vi "ColourSensorProcess.vi"(8 "error in (no error)":errorcluster, 9 "I2C Ref Out":T1={"myRIO Reference"={"myRIO Model"=enum."myRIO-1900", "myRIO Hardware Reference"={"Generic FPGA Reference"=refnum, "Allow multiple opens"=TRUE}}, "I2C Channels Enum"=enum."A/I2C", "I2C Configuration"={"I2C Transfer Rate"=enum."Fast mode (400 kbps)"}}, 10 "Just the ascending angles":dbl[](array[numeric])=[0.0, 0.49085178039801924, 0.49085178039801924, 0.4969686048790533, 0.5016040541891205, 0.5028432109278608, 0.5084893240796899, 0.5084893240796899, 0.5084893240796899, 0.5084893240796899, 0.5115561271703055, 0.5123894603107377, 0.5139196809985338, 0.5139196809985338, 0.5139196809985338, 0.5139196809985338, 0.5139196809985338, 0.5139196809985338, 0.5139196809985338, 0.515549007458979, 0.515549007458979, 0.515549007458979, 0.515549007458979, 0.515549007458979, 0.515549007458979, 0.5172873803276212, 0.5172873803276212, 0.5191461142465229, 0.5209097808482157, 0.5209097808482157, 0.5211381434841182, 0.5224034317165288, 0.5227890853804023, 0.5227890853804023, 0.5227890853804023, 0.5227890853804023, 0.5227890853804023, 0.5227890853804023, 0.5241796287829132, 0.5241796287829132, 0.5241796287829132, 0.5241796287829132, 0.5241796287829132, 0.5247957716501074, 0.5260664189967634, 0.5260664189967634, 0.5280744484263596, 0.5280744484263596, 0.5280744484263596, 0.5280744484263596, 0.5290304710796486, 0.5290304710796486, 0.5302157727766299, 0.5302157727766299, 0.5302157727766299, 0.5302157727766299, 0.5302157727766299, 0.5302157727766299, 0.5337081916392615, 0.5358112379604637, 0.5404195002705842, 0.5434775947130435, 0.5448639154515437, 0.5448639154515437, 0.5467888408892474, 0.8058034940839864, 0.8066715494215095, 0.8066715494215095, 0.8066715494215095, 0.8066715494215095, 0.8066715494215095, 0.8066715494215095, 0.8066715494215095, 0.8076167287241673, 0.8076167287241673, 0.8076167287241673, 0.8076167287241673, 0.8076167287241673, 0.8076167287241673, 0.8086497862079112, 0.8086497862079112, 0.8086497862079112, 0.8253768505207384, 0.8253768505207384, 0.8253768505207384, 0.8253768505207384, 0.8253768505207384, 0.8253768505207384, 0.8253768505207384, 0.8270407424960368, 0.8270407424960368, 0.8270407424960368, 0.8270407424960368, 0.8270407424960368, 0.8270407424960368, 0.8270407424960368, 0.8288490587889792, 0.8288490587889792, 0.8288490587889792, 0.8288490587889792, 0.8288490587889792, 0.8288490587889792, 0.8288490587889792, 0.8288490587889792, 0.8288490587889792, 0.8288490587889792, 0.8288490587889792, 0.8288490587889792, 0.8288490587889792, 0.8288490587889792, 0.8288490587889792, 0.8288490587889792, 0.8288490587889792, 0.8288490587889792, 0.8288490587889792, 0.8288490587889792, 0.8288490587889792, 0.8288490587889792, 0.8288490587889792, 0.8288490587889792, 0.8308214428190254, 0.8308214428190254, 0.8308214428190254, 0.8329812666744317, 0.8329812666744317, 0.8329812666744317, 0.8347407956504183, 0.8348627319990397, 0.8351908590380576, 0.8351908590380576, 0.8355233647892368, 0.8355233647892368, 0.8359878721668329, 0.8359878721668329, 0.8359878721668329, 0.8361009389134209, 0.8362018674556699, 0.8366353308008672, 0.8366353308008672, 0.8367125926410904, 0.8369653093402846, 0.8370239821610109, 0.8372995618556213, 0.8373391705219767, 0.8373391705219767, 0.8376381718486057, 0.8376582276036019, 0.8376582276036019, 0.83798122500839, 0.83798122500839, 0.83798122500839, 0.83798122500839, 0.83798122500839, 0.83798122500839, 0.83798122500839, 0.83798122500839, 0.83798122500839, 0.83798122500839, 0.8383082361151116, 0.8383082361151116, 0.8383082361151116, 0.8383082361151116, 0.8383288092835823, 0.8386393361341747, 0.8386810149571406, 0.8389746021650794, 0.8393996637734166, 0.8396579504659081, 0.8398896196381795, 0.8398896196381795, 0.8398896196381795, 0.8402212212619267, 0.8402212212619267, 0.8403589379188695, 0.8403589379188695, 0.8405568793256272, 0.8405568793256272, 0.8405568793256272, 0.8405568793256272, 0.8412406658776183, 1.2662854435927842, 1.271020256694917, 1.2760662215855192, 1.2801238458816968, 1.281104755549737, 1.2866624282690307, 1.2901185509887085, 1.2924966677897853, 1.2924966677897853, 1.2924966677897853, 1.2936356194613072, 1.2949904282063742, 1.2963477398940586, 1.2971370057128062, 1.2984560728064871, 1.2994010459932608, 1.299849476456476, 1.300770710650036, 1.301323676862733, 1.3016288340091962, 1.3022168962760163, 1.3030472727742226, 1.3045442776439713, 1.3045442776439713, 1.3045442776439713, 1.3045442776439713, 1.3053659701459766, 1.3059789968891078, 1.3061265548045191, 1.3061265548045191, 1.3068326031691921, 1.3078015951139772, 1.3084658261687312, 1.3084658261687312, 1.3084658261687312, 1.3084658261687312, 1.3090828243936916, 1.3090828243936916, 1.3096574544123287, 1.312544106983858, 1.3130251845606, 1.3130251845606, 1.3130251845606, 1.3148531907902146, 1.3156139361740782, 1.316788563668303, 1.317122230656254, 1.3177206746302943, 1.3177206746302943, 1.3188410326762603, 1.3193522365168788, 1.3195807383028326, 1.321209401357912, 1.321209401357912, 1.3213831029368495, 1.321544185409683, 1.3216939757021517, 1.3216939757021517, 1.3236198650089266, 1.3236990227701797, 1.3258176636680326, 1.3279009939872919, 1.3280598123771263, 1.329949871553485, 1.330262078848992, 1.330262078848992, 1.330262078848992, 1.3324254970081457, 1.3324254970081457, 1.3407101796026626, 1.3439974787410107], 11 "All colours in ascending angles: R/G/B/num/angle":dbl[][](array[numeric])=[[0.0, 0.0, 0.0, 3.0, 0.0], [31.0, 58.0, 26.0, 2.0, 0.49085178039801924], [31.0, 58.0, 26.0, 2.0, 0.49085178039801924], [32.0, 59.0, 27.0, 2.0, 0.4969686048790533], [34.0, 62.0, 29.0, 2.0, 0.5016040541891205], [33.0, 60.0, 27.0, 2.0, 0.5028432109278608], [34.0, 61.0, 28.0, 2.0, 0.5084893240796899], [34.0, 61.0, 28.0, 2.0, 0.5084893240796899], [34.0, 61.0, 29.0, 2.0, 0.5084893240796899], [34.0, 61.0, 28.0, 2.0, 0.5084893240796899], [32.0, 57.0, 26.0, 2.0, 0.5115561271703055], [36.0, 64.0, 30.0, 2.0, 0.5123894603107377], [35.0, 62.0, 29.0, 2.0, 0.5139196809985338], [35.0, 62.0, 29.0, 2.0, 0.5139196809985338], [35.0, 62.0, 29.0, 2.0, 0.5139196809985338], [35.0, 62.0, 29.0, 2.0, 0.5139196809985338], [35.0, 62.0, 29.0, 2.0, 0.5139196809985338], [35.0, 62.0, 29.0, 2.0, 0.5139196809985338], [35.0, 62.0, 29.0, 2.0, 0.5139196809985338], [34.0, 60.0, 28.0, 2.0, 0.515549007458979], [34.0, 60.0, 28.0, 2.0, 0.515549007458979], [34.0, 60.0, 28.0, 2.0, 0.515549007458979], [34.0, 60.0, 28.0, 2.0, 0.515549007458979], [34.0, 60.0, 28.0, 2.0, 0.515549007458979], [34.0, 60.0, 28.0, 2.0, 0.515549007458979], [33.0, 58.0, 27.0, 2.0, 0.5172873803276212], [33.0, 58.0, 27.0, 2.0, 0.5172873803276212], [36.0, 63.0, 30.0, 2.0, 0.5191461142465229], [35.0, 61.0, 29.0, 2.0, 0.5209097808482157], [35.0, 61.0, 28.0, 2.0, 0.5209097808482157], [31.0, 54.0, 25.0, 2.0, 0.5211381434841182], [38.0, 66.0, 31.0, 2.0, 0.5224034317165288], [34.0, 59.0, 28.0, 2.0, 0.5227890853804023], [34.0, 59.0, 28.0, 2.0, 0.5227890853804023], [34.0, 59.0, 28.0, 2.0, 0.5227890853804023], [34.0, 59.0, 28.0, 2.0, 0.5227890853804023], [34.0, 59.0, 28.0, 2.0, 0.5227890853804023], [34.0, 59.0, 27.0, 2.0, 0.5227890853804023], [37.0, 64.0, 30.0, 2.0, 0.5241796287829132], [37.0, 64.0, 31.0, 2.0, 0.5241796287829132], [37.0, 64.0, 30.0, 2.0, 0.5241796287829132], [37.0, 64.0, 30.0, 2.0, 0.5241796287829132], [37.0, 64.0, 31.0, 2.0, 0.5241796287829132], [33.0, 57.0, 27.0, 2.0, 0.5247957716501074], [36.0, 62.0, 30.0, 2.0, 0.5260664189967634], [36.0, 62.0, 29.0, 2.0, 0.5260664189967634], [35.0, 60.0, 28.0, 2.0, 0.5280744484263596], [35.0, 60.0, 28.0, 2.0, 0.5280744484263596], [35.0, 60.0, 28.0, 2.0, 0.5280744484263596], [35.0, 60.0, 28.0, 2.0, 0.5280744484263596], [38.0, 65.0, 31.0, 2.0, 0.5290304710796486], [38.0, 65.0, 31.0, 2.0, 0.5290304710796486], [34.0, 58.0, 28.0, 2.0, 0.5302157727766299], [34.0, 58.0, 28.0, 2.0, 0.5302157727766299], [34.0, 58.0, 28.0, 2.0, 0.5302157727766299], [34.0, 58.0, 28.0, 2.0, 0.5302157727766299], [34.0, 58.0, 28.0, 2.0, 0.5302157727766299], [34.0, 58.0, 28.0, 2.0, 0.5302157727766299], [39.0, 66.0, 32.0, 2.0, 0.5337081916392615], [38.0, 64.0, 31.0, 2.0, 0.5358112379604637], [30.0, 50.0, 24.0, 2.0, 0.5404195002705842], [29.0, 48.0, 23.0, 2.0, 0.5434775947130435], [40.0, 66.0, 33.0, 2.0, 0.5448639154515437], [40.0, 66.0, 32.0, 2.0, 0.5448639154515437], [28.0, 46.0, 22.0, 2.0, 0.5467888408892474], [25.0, 24.0, 16.0, 4.0, 0.8058034940839864], [24.0, 23.0, 15.0, 4.0, 0.8066715494215095], [24.0, 23.0, 15.0, 4.0, 0.8066715494215095], [24.0, 23.0, 15.0, 4.0, 0.8066715494215095], [24.0, 23.0, 15.0, 4.0, 0.8066715494215095], [24.0, 23.0, 15.0, 4.0, 0.8066715494215095], [24.0, 23.0, 15.0, 4.0, 0.8066715494215095], [24.0, 23.0, 15.0, 4.0, 0.8066715494215095], [23.0, 22.0, 14.0, 4.0, 0.8076167287241673], [23.0, 22.0, 14.0, 4.0, 0.8076167287241673], [23.0, 22.0, 14.0, 4.0, 0.8076167287241673], [23.0, 22.0, 14.0, 4.0, 0.8076167287241673], [23.0, 22.0, 14.0, 4.0, 0.8076167287241673], [23.0, 22.0, 14.0, 4.0, 0.8076167287241673], [22.0, 21.0, 14.0, 4.0, 0.8086497862079112], [22.0, 21.0, 14.0, 4.0, 0.8086497862079112], [22.0, 21.0, 14.0, 4.0, 0.8086497862079112], [26.0, 24.0, 16.0, 4.0, 0.8253768505207384], [26.0, 24.0, 16.0, 4.0, 0.8253768505207384], [26.0, 24.0, 16.0, 4.0, 0.8253768505207384], [26.0, 24.0, 16.0, 4.0, 0.8253768505207384], [26.0, 24.0, 16.0, 4.0, 0.8253768505207384], [26.0, 24.0, 16.0, 4.0, 0.8253768505207384], [26.0, 24.0, 16.0, 4.0, 0.8253768505207384], [25.0, 23.0, 15.0, 4.0, 0.8270407424960368], [25.0, 23.0, 16.0, 4.0, 0.8270407424960368], [25.0, 23.0, 16.0, 4.0, 0.8270407424960368], [25.0, 23.0, 16.0, 4.0, 0.8270407424960368], [25.0, 23.0, 16.0, 4.0, 0.8270407424960368], [25.0, 23.0, 15.0, 4.0, 0.8270407424960368], [25.0, 23.0, 16.0, 4.0, 0.8270407424960368], [24.0, 22.0, 15.0, 4.0, 0.8288490587889792], [24.0, 22.0, 14.0, 4.0, 0.8288490587889792], [24.0, 22.0, 15.0, 4.0, 0.8288490587889792], [24.0, 22.0, 14.0, 4.0, 0.8288490587889792], [24.0, 22.0, 15.0, 4.0, 0.8288490587889792], [24.0, 22.0, 15.0, 4.0, 0.8288490587889792], [24.0, 22.0, 15.0, 4.0, 0.8288490587889792], [24.0, 22.0, 15.0, 4.0, 0.8288490587889792], [24.0, 22.0, 15.0, 4.0, 0.8288490587889792], [24.0, 22.0, 14.0, 4.0, 0.8288490587889792], [24.0, 22.0, 14.0, 4.0, 0.8288490587889792], [24.0, 22.0, 15.0, 4.0, 0.8288490587889792], [24.0, 22.0, 14.0, 4.0, 0.8288490587889792], [24.0, 22.0, 15.0, 4.0, 0.8288490587889792], [24.0, 22.0, 15.0, 4.0, 0.8288490587889792], [24.0, 22.0, 15.0, 4.0, 0.8288490587889792], [24.0, 22.0, 15.0, 4.0, 0.8288490587889792], [24.0, 22.0, 15.0, 4.0, 0.8288490587889792], [24.0, 22.0, 15.0, 4.0, 0.8288490587889792], [24.0, 22.0, 15.0, 4.0, 0.8288490587889792], [24.0, 22.0, 15.0, 4.0, 0.8288490587889792], [24.0, 22.0, 14.0, 4.0, 0.8288490587889792], [24.0, 22.0, 15.0, 4.0, 0.8288490587889792], [24.0, 22.0, 14.0, 4.0, 0.8288490587889792], [23.0, 21.0, 14.0, 4.0, 0.8308214428190254], [23.0, 21.0, 14.0, 4.0, 0.8308214428190254], [23.0, 21.0, 14.0, 4.0, 0.8308214428190254], [22.0, 20.0, 13.0, 4.0, 0.8329812666744317], [22.0, 20.0, 13.0, 4.0, 0.8329812666744317], [22.0, 20.0, 13.0, 4.0, 0.8329812666744317], [170.0, 154.0, 60.0, 3.0, 0.8347407956504183], [159.0, 144.0, 58.0, 3.0, 0.8348627319990397], [158.0, 143.0, 58.0, 3.0, 0.8351908590380576], [158.0, 143.0, 58.0, 3.0, 0.8351908590380576], [157.0, 142.0, 57.0, 3.0, 0.8355233647892368], [157.0, 142.0, 56.0, 3.0, 0.8355233647892368], [166.0, 150.0, 61.0, 3.0, 0.8359878721668329], [166.0, 150.0, 60.0, 3.0, 0.8359878721668329], [166.0, 150.0, 60.0, 3.0, 0.8359878721668329], [176.0, 159.0, 65.0, 3.0, 0.8361009389134209], [155.0, 140.0, 56.0, 3.0, 0.8362018674556699], [164.0, 148.0, 60.0, 3.0, 0.8366353308008672], [164.0, 148.0, 59.0, 3.0, 0.8366353308008672], [174.0, 157.0, 63.0, 3.0, 0.8367125926410904], [163.0, 147.0, 59.0, 3.0, 0.8369653093402846], [173.0, 156.0, 63.0, 3.0, 0.8370239821610109], [162.0, 146.0, 59.0, 3.0, 0.8372995618556213], [172.0, 155.0, 62.0, 3.0, 0.8373391705219767], [172.0, 155.0, 62.0, 3.0, 0.8373391705219767], [161.0, 145.0, 58.0, 3.0, 0.8376381718486057], [171.0, 154.0, 62.0, 3.0, 0.8376582276036019], [171.0, 154.0, 62.0, 3.0, 0.8376582276036019], [170.0, 153.0, 62.0, 3.0, 0.83798122500839], [160.0, 144.0, 58.0, 3.0, 0.83798122500839], [160.0, 144.0, 58.0, 3.0, 0.83798122500839], [160.0, 144.0, 58.0, 3.0, 0.83798122500839], [170.0, 153.0, 61.0, 3.0, 0.83798122500839], [170.0, 153.0, 62.0, 3.0, 0.83798122500839], [170.0, 153.0, 60.0, 3.0, 0.83798122500839], [170.0, 153.0, 60.0, 3.0, 0.83798122500839], [170.0, 153.0, 60.0, 3.0, 0.83798122500839], [170.0, 153.0, 60.0, 3.0, 0.83798122500839], [169.0, 152.0, 61.0, 3.0, 0.8383082361151116], [169.0, 152.0, 60.0, 3.0, 0.8383082361151116], [169.0, 152.0, 61.0, 3.0, 0.8383082361151116], [169.0, 152.0, 60.0, 3.0, 0.8383082361151116], [159.0, 143.0, 58.0, 3.0, 0.8383288092835823], [168.0, 151.0, 58.0, 3.0, 0.8386393361341747], [158.0, 142.0, 58.0, 3.0, 0.8386810149571406], [167.0, 150.0, 60.0, 3.0, 0.8389746021650794], [156.0, 140.0, 56.0, 3.0, 0.8393996637734166], [165.0, 148.0, 59.0, 3.0, 0.8396579504659081], [174.0, 156.0, 63.0, 3.0, 0.8398896196381795], [174.0, 156.0, 63.0, 3.0, 0.8398896196381795], [174.0, 156.0, 63.0, 3.0, 0.8398896196381795], [173.0, 155.0, 62.0, 3.0, 0.8402212212619267], [173.0, 155.0, 62.0, 3.0, 0.8402212212619267], [163.0, 146.0, 59.0, 3.0, 0.8403589379188695], [163.0, 146.0, 59.0, 3.0, 0.8403589379188695], [172.0, 154.0, 62.0, 3.0, 0.8405568793256272], [172.0, 154.0, 62.0, 3.0, 0.8405568793256272], [172.0, 154.0, 63.0, 3.0, 0.8405568793256272], [172.0, 154.0, 62.0, 3.0, 0.8405568793256272], [170.0, 152.0, 61.0, 3.0, 0.8412406658776183], [105.0, 33.0, 26.0, 1.0, 1.2662854435927842], [110.0, 34.0, 28.0, 1.0, 1.271020256694917], [112.0, 34.0, 29.0, 1.0, 1.2760662215855192], [117.0, 35.0, 30.0, 1.0, 1.2801238458816968], [104.0, 31.0, 25.0, 1.0, 1.281104755549737], [113.0, 33.0, 28.0, 1.0, 1.2866624282690307], [111.0, 32.0, 27.0, 1.0, 1.2901185509887085], [112.0, 32.0, 27.0, 1.0, 1.2924966677897853], [112.0, 32.0, 27.0, 1.0, 1.2924966677897853], [105.0, 30.0, 26.0, 1.0, 1.2924966677897853], [116.0, 33.0, 28.0, 1.0, 1.2936356194613072], [106.0, 30.0, 25.0, 1.0, 1.2949904282063742], [103.0, 29.0, 25.0, 1.0, 1.2963477398940586], [114.0, 32.0, 28.0, 1.0, 1.2971370057128062], [111.0, 31.0, 26.0, 1.0, 1.2984560728064871], [115.0, 32.0, 27.0, 1.0, 1.2994010459932608], [108.0, 30.0, 25.0, 1.0, 1.299849476456476], [112.0, 31.0, 26.0, 1.0, 1.300770710650036], [105.0, 29.0, 24.0, 1.0, 1.301323676862733], [116.0, 32.0, 27.0, 1.0, 1.3016288340091962], [109.0, 30.0, 26.0, 1.0, 1.3022168962760163], [113.0, 31.0, 27.0, 1.0, 1.3030472727742226], [110.0, 30.0, 26.0, 1.0, 1.3045442776439713], [110.0, 30.0, 26.0, 1.0, 1.3045442776439713], [110.0, 30.0, 26.0, 1.0, 1.3045442776439713], [110.0, 30.0, 26.0, 1.0, 1.3045442776439713], [103.0, 28.0, 24.0, 1.0, 1.3053659701459766], [118.0, 32.0, 28.0, 1.0, 1.3059789968891078], [107.0, 29.0, 24.0, 1.0, 1.3061265548045191], [107.0, 29.0, 24.0, 1.0, 1.3061265548045191], [111.0, 30.0, 26.0, 1.0, 1.3068326031691921], [104.0, 28.0, 24.0, 1.0, 1.3078015951139772], [108.0, 29.0, 25.0, 1.0, 1.3084658261687312], [108.0, 29.0, 25.0, 1.0, 1.3084658261687312], [108.0, 29.0, 25.0, 1.0, 1.3084658261687312], [108.0, 29.0, 25.0, 1.0, 1.3084658261687312], [112.0, 30.0, 26.0, 1.0, 1.3090828243936916], [112.0, 30.0, 26.0, 1.0, 1.3090828243936916], [116.0, 31.0, 27.0, 1.0, 1.3096574544123287], [106.0, 28.0, 24.0, 1.0, 1.312544106983858], [110.0, 29.0, 25.0, 1.0, 1.3130251845606], [110.0, 29.0, 25.0, 1.0, 1.3130251845606], [110.0, 29.0, 25.0, 1.0, 1.3130251845606], [107.0, 28.0, 24.0, 1.0, 1.3148531907902146], [115.0, 30.0, 26.0, 1.0, 1.3156139361740782], [104.0, 27.0, 23.0, 1.0, 1.316788563668303], [108.0, 28.0, 24.0, 1.0, 1.317122230656254], [116.0, 30.0, 26.0, 1.0, 1.3177206746302943], [116.0, 30.0, 26.0, 1.0, 1.3177206746302943], [101.0, 26.0, 23.0, 1.0, 1.3188410326762603], [109.0, 28.0, 24.0, 1.0, 1.3193522365168788], [113.0, 29.0, 26.0, 1.0, 1.3195807383028326], [102.0, 26.0, 23.0, 1.0, 1.321209401357912], [102.0, 26.0, 23.0, 1.0, 1.321209401357912], [106.0, 27.0, 23.0, 1.0, 1.3213831029368495], [110.0, 28.0, 24.0, 1.0, 1.321544185409683], [114.0, 29.0, 26.0, 1.0, 1.3216939757021517], [114.0, 29.0, 25.0, 1.0, 1.3216939757021517], [107.0, 27.0, 23.0, 1.0, 1.3236198650089266], [111.0, 28.0, 24.0, 1.0, 1.3236990227701797], [104.0, 26.0, 22.0, 1.0, 1.3258176636680326], [113.0, 28.0, 25.0, 1.0, 1.3279009939872919], [105.0, 26.0, 23.0, 1.0, 1.3280598123771263], [114.0, 28.0, 25.0, 1.0, 1.329949871553485], [106.0, 26.0, 22.0, 1.0, 1.330262078848992], [106.0, 26.0, 23.0, 1.0, 1.330262078848992], [106.0, 26.0, 22.0, 1.0, 1.330262078848992], [107.0, 26.0, 23.0, 1.0, 1.3324254970081457], [107.0, 26.0, 23.0, 1.0, 1.3324254970081457], [111.0, 26.0, 24.0, 1.0, 1.3407101796026626], [104.0, 24.0, 21.0, 1.0, 1.3439974787410107]]) -> (1 "?":i32=76, 2 "Numeric":dbl=4.0, 3 "lower limit":dbl=64.0, 4 "upper limit":dbl=180.0, 5 "Angle":dbl=0.8288490587889792)   [LabVIEW 2017]
uses:
  <vilib>/myRIO/Instrument Drivers/Onboard IO/I2C/typedefs/I2C Reference.ctl
  <vilib>/myRIO/Common/Instrument Driver Framework/Utilities/typedefs/myRIO Generic Hardware Reference.ctl
  <vilib>/myRIO/Common/Instrument Driver Framework/Utilities/typedefs/Hardware Version Enum.ctl
  <vilib>/myRIO/Common/Instrument Driver Framework/Utilities/typedefs/myRIO v1.0 Reference.ctl
  <vilib>/myRIO/Common/Instrument Driver Framework/Utilities/typedefs/Generic FPGA Reference.ctl
  <vilib>/myRIO/Common/Instrument Driver Framework/myRIO v1.0/I2C/typedefs/I2C Channels Enum.ctl
  <vilib>/myRIO/Instrument Drivers/Onboard IO/I2C/typedefs/I2C Configuration.ctl
  <vilib>/myRIO/Instrument Drivers/Onboard IO/I2C/typedefs/I2C Transfer Rate.ctl
  <vilib>/Analysis/baseanly.llb/Unimode.vi
  <vilib>/Analysis/NI_AALBase.lvlib
  <vilib>/myRIO/Instrument Drivers/Onboard IO/I2C/I2C.lvlib
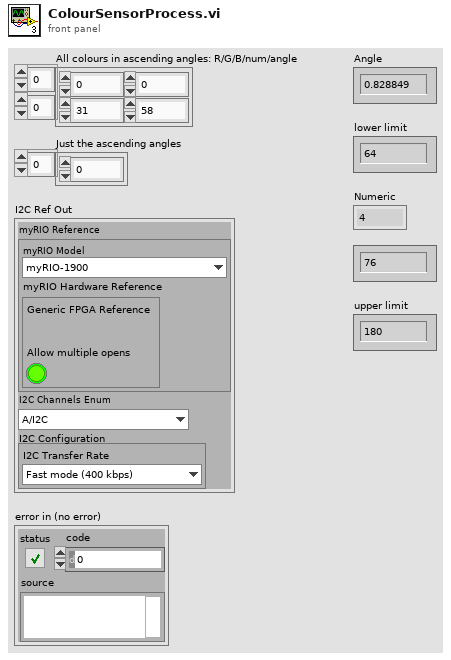
[diagram p1: front panel]
types:
  T1 = typedef "I2C.lvlib/I2C Reference.ctl" = cluster{"myRIO Reference":T2, "I2C Channels Enum":T6, "I2C Configuration":T7}
  T2 = typedef "myRIO Generic Hardware Reference.ctl" = cluster{"myRIO Model":T3, "myRIO Hardware Reference":T4}
  T3 = typedef "Hardware Version Enum.ctl" = enum16{"Unknown", "myRIO-1900", "myRIO-1950", "roboRIO", "NI ELVIS RIO CM"}
  T4 = typedef "myRIO v1.0 Reference.ctl" = cluster{"Generic FPGA Reference":T5, "Allow multiple opens":bool}
  T5 = typedef "Generic FPGA Reference.ctl" = refnum<k20>
  T6 = typedef "I2C Channels Enum.ctl" = enum16{"Not Connected", "A/I2C", "B/I2C", "I2C/I2C"}
  T7 = typedef "I2C.lvlib/I2C Configuration.ctl" = cluster{"I2C Transfer Rate":T8}
  T8 = typedef "I2C.lvlib/I2C Transfer Rate.ctl" = enum16{"Standard mode (100 kbps)", "Fast mode (400 kbps)"}
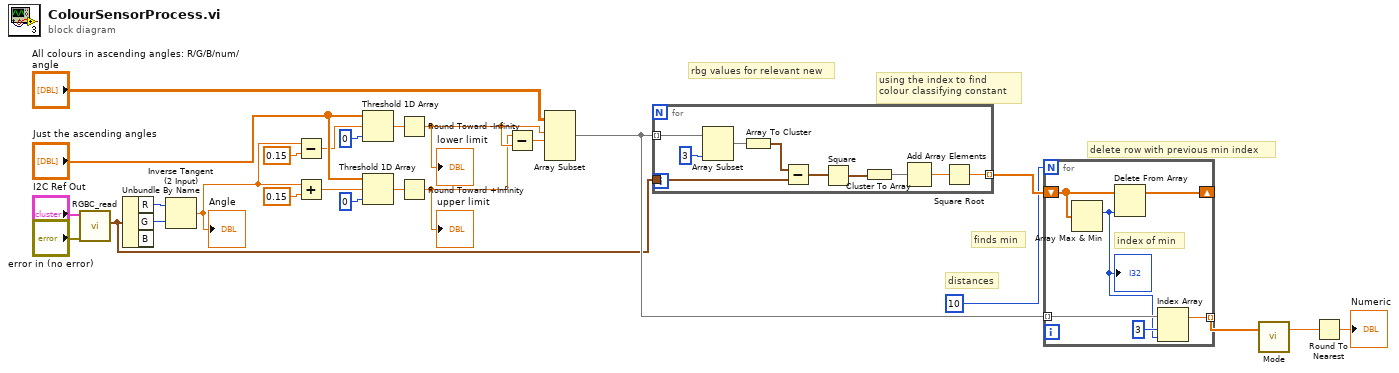
[diagram p0: block diagram]
diagram:
  # "finds min"
  # "delete row with previous min index"
  # "distances"
  # "rbg values for relevant new"
  # "using the index to find \ncolour classifying constant"
  n1 = call "RGBC_read.vi"("error in (no error)"="error in (no error)", "I2C Ref In"="I2C Ref Out") -> ("RGB"=w19:cluster{"R":u8, "G":u8, "B":u8})  [unwired: 7 in, 2 out]
  n2 = Unbundle By Name(w19) -> ("R"=w15:u8, "G"=w16:u8)  [unwired: 1 out]
  n3 = Inverse Tangent (2 Input)(1:w16, 2:w15) -> (0:w6:dbl)
  "Angle" <- w6
  n4 = Subtract(x=w6, y=0.15) -> (x-y=w7:dbl)
  n5 = Add(x=w6, y=0.15) -> (x+y=w4:dbl)
  n6 = Threshold 1D Array(1:0 ("start index (0)"), 2:w7, 3:"Just the ascending angles") -> (0:w9:dbl)
  n7 = Threshold 1D Array(1:0 ("start index (0)"), 2:w4, 3:"Just the ascending angles") -> (0:w8:dbl)
  n8 = Round Toward -Infinity(1:w9) -> (0:w12:dbl)
  "lower limit" <- w12
  n9 = Round Toward +Infinity(x=w8) -> (ceil(x): smallest int >= x=w10:dbl)
  "upper limit" <- w10
  n10 = Subtract(x=w10, y=w12) -> (x-y=w11:dbl)
  n11 = Array Subset(array="All colours in ascending angles: R/G/B/num/angle", index (row)=w12, length (row)=w11) -> (w20:dbl[][])  [unwired: 2 in]
  n12 = for {
    tunnel: w20 -> [w33] mode=indexing
    tunnel: [w35] -> w25 mode=indexing
    tunnel: w19 -> [w30]
    n13 = Array Subset(array=w33, length=3) -> (w31:dbl[])  [unwired: 1 in]
    n14 = Array To Cluster(array=w31) -> (cluster=w29:cluster{"[0]":dbl, "[1]":dbl, "[2]":dbl})
    n15 = Subtract(x=w29, y=w30) -> (x-y=w34:cluster{dbl, dbl, dbl})
    n16 = Square(x=w34) -> (x^2=w28:cluster{dbl, dbl, dbl})
    n17 = Cluster To Array(cluster=w28) -> (array=w27:dbl[])
    n18 = Add Array Elements(numeric array=w27) -> (sum=w26:dbl)
    n19 = Square Root(x=w26) -> (sqrt(x)=w35:dbl)
  }
  n20 = for {
    N: 10 -> [_]
    tunnel: w20 -> [w39] mode=indexing
    tunnel: [w40] -> w21 mode=indexing
    shift-right: [w41] -> _
    shift-left: w25 -> [w37]
    # "index of min"
    n21 = Array Max & Min(array=w37) -> (max index (indices)=w36:i32)  [unwired: 3 out]
    "?" <- w36
    n22 = Delete From Array(array=w37, index=w36) -> (array with subset deleted=w41:dbl[])  [unwired: 1 in, 1 out]
    n23 = Index Array(array=w39, index #1=3 ("disabled index (row)"), index #2=w36) -> (element #1=w40:dbl)  [unwired: 1 out]
  }
  n24 = call-poly <vilib>:"Mode.vi"("X"=w21) -> ("mode"=w23:dbl)  [unwired: 1 in, 1 out]
  n25 = Round To Nearest(number=w23) -> (nearest integer value=→"Numeric":dbl)
